vi "2022_version.vi"() -> ()   [LabVIEW 2022 SP3]
panel:
  out "output cluster":cluster{"current speed":dbl, "command":string}
  in  "input":cluster{"current speed":dbl, "command":string}
  out "test pic":picture
  in  "image_path":path
  out "return value":string
  in  "module path":path
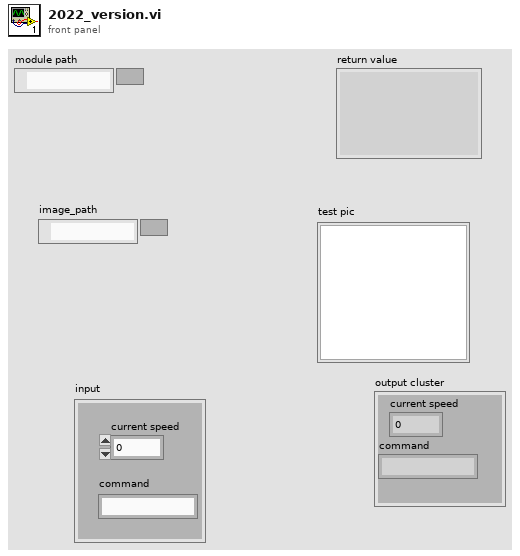
[diagram p1: front panel]
types:
  T1 = typedef "imagedata.ctl" = cluster{"image type":i32, "image depth":i32, "image":u8[], "mask":u8[], "colors":u32[], "Rectangle":cluster{"left":i16, "top":i16, "right":i16, "bottom":i16}}
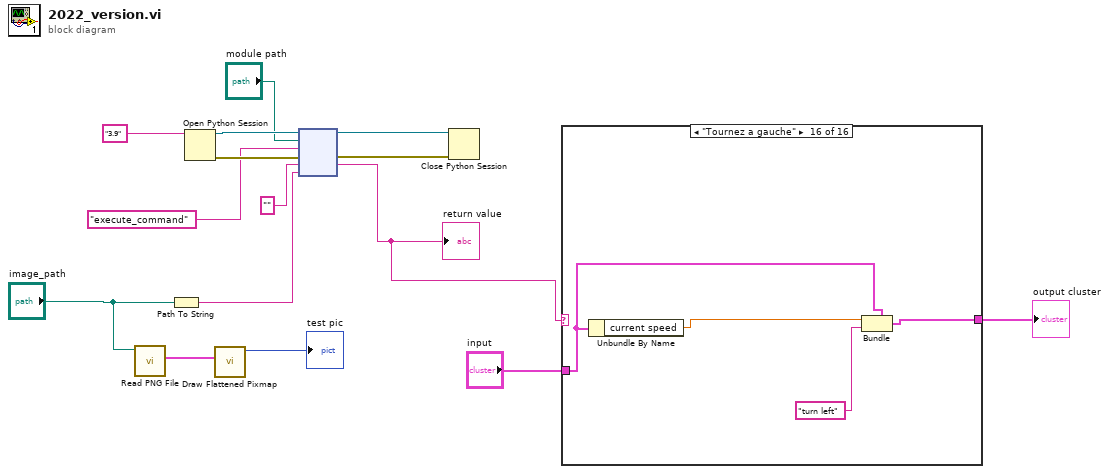
[diagram p0: block diagram]
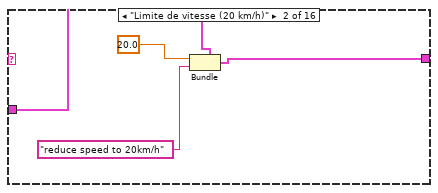
[diagram p3: hidden frame]
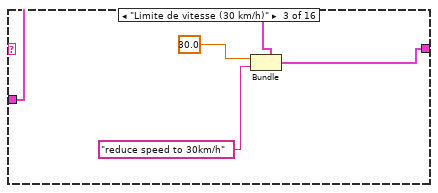
[diagram p4: hidden frame]
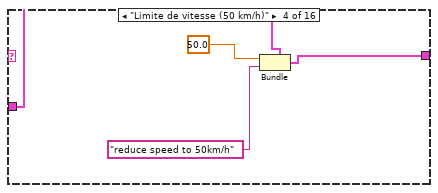
[diagram p5: hidden frame]
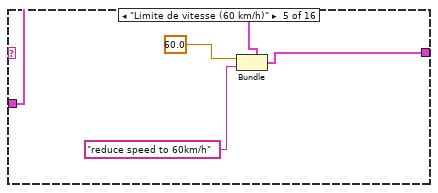
[diagram p6: hidden frame]
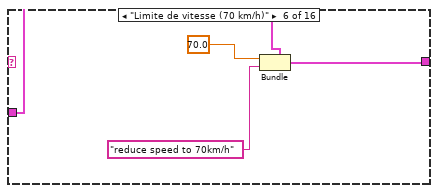
[diagram p7: hidden frame]
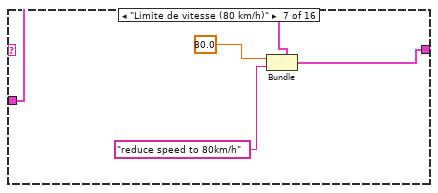
[diagram p8: hidden frame]
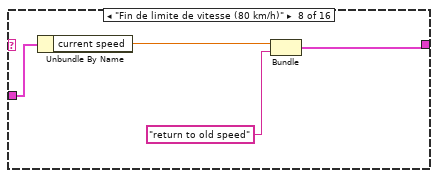
[diagram p9: hidden frame]
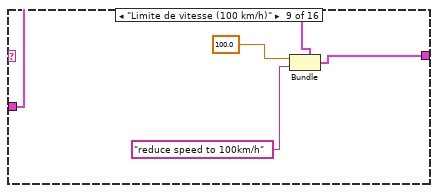
[diagram p10: hidden frame]
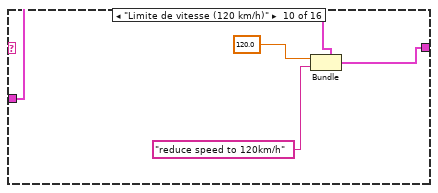
[diagram p11: hidden frame]
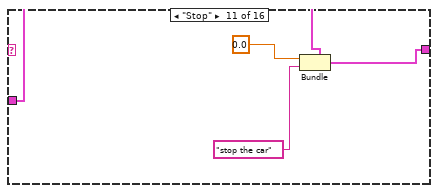
[diagram p12: hidden frame]
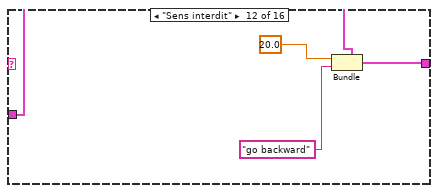
[diagram p13: hidden frame]
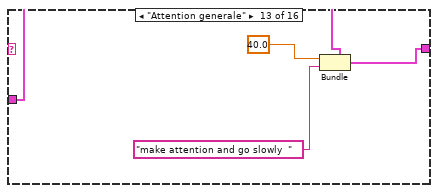
[diagram p14: hidden frame]
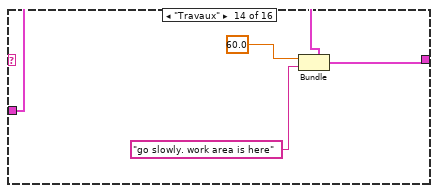
[diagram p15: hidden frame]
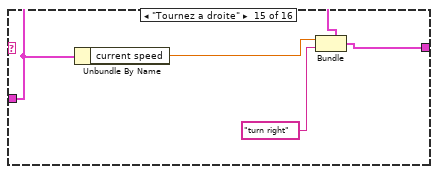
[diagram p16: hidden frame]
diagram:
  n1 = call <vilib>:"Read PNG File.vi"("path to PNG file"="image_path") -> ("image data"=w5:T1)  [unwired: 8 in, 2 out]
  n2 = Path To String(path="image_path") -> (string=w7:string)
  n3 = Open Python Session(python version="3.9" ("Python version")) -> (session out=w15:refnum<k35>, error out=w13:errorcluster)  [unwired: 2 in]
  n4 = call <vilib>:"Draw Flattened Pixmap.vi"("image data"=w5) -> ("new picture"=→"test pic":picture)  [unwired: 8 in]
  n5 = node(w15, "module path", "execute_command" ("function name"), w13, "", w7) -> (w14:refnum<k35>, w12:errorcluster, w3:string)  [unwired: 1 in, 2 out]
  "return value" <- w3
  n6 = Close Python Session(session in=w14, error in=w12) -> ()  [unwired: 1 out]
  n7 = case shown="\"Tournez a gauche\"" w3 {
    tunnel: "input" -> [w16 w20 w22 w26 w30 w34 w38 w43 w46 w49 w54 w58 w62 w66 w70 w74]
    tunnel: [w16 w17 w21 w25 w29 w33 w37 w41 w45 w50 w53 w57 w61 w65 w71 w75] -> w1
    frame "False", Default {
    }
    frame "Limite de vitesse (20 km/h)" {
      n8 = Bundle(cluster=w20, "current speed"=20.0, "command"="reduce speed to 20km/h") -> (w17:cluster{"current speed":dbl, "command":string})
    }
    frame "Limite de vitesse (30 km/h)" {
      n9 = Bundle(cluster=w22, "current speed"=30.0, "command"="reduce speed to 30km/h") -> (w21:cluster{"current speed":dbl, "command":string})
    }
    frame "Limite de vitesse (50 km/h)" {
      n10 = Bundle(cluster=w26, "current speed"=50.0, "command"="reduce speed to 50km/h") -> (w25:cluster{"current speed":dbl, "command":string})
    }
    frame "Limite de vitesse (60 km/h)" {
      n11 = Bundle(cluster=w30, "current speed"=60.0, "command"="reduce speed to 60km/h") -> (w29:cluster{"current speed":dbl, "command":string})
    }
    frame "Limite de vitesse (70 km/h)" {
      n12 = Bundle(cluster=w34, "current speed"=70.0, "command"="reduce speed to 70km/h") -> (w33:cluster{"current speed":dbl, "command":string})
    }
    frame "Limite de vitesse (80 km/h)" {
      n13 = Bundle(cluster=w38, "current speed"=80.0, "command"="reduce speed to 80km/h") -> (w37:cluster{"current speed":dbl, "command":string})
    }
    frame "Fin de limite de vitesse (80 km/h)" {
      n14 = Unbundle By Name(w43) -> ("current speed"=w42:dbl)
      n15 = Bundle("current speed"=w42, "command"="return to old speed") -> (w41:cluster{"current speed":dbl, "command":string})  [unwired: 1 in]
    }
    frame "Limite de vitesse (100 km/h)" {
      n16 = Bundle(cluster=w46, "current speed"=100.0, "command"="reduce speed to 100km/h") -> (w45:cluster{"current speed":dbl, "command":string})
    }
    frame "Limite de vitesse (120 km/h)" {
      n17 = Bundle(cluster=w49, "current speed"=120.0, "command"="reduce speed to 120km/h") -> (w50:cluster{"current speed":dbl, "command":string})
    }
    frame "Stop" {
      n18 = Bundle(cluster=w54, "current speed"=0.0, "command"="stop the car") -> (w53:cluster{"current speed":dbl, "command":string})
    }
    frame "Sens interdit" {
      n19 = Bundle(cluster=w58, "current speed"=20.0, "command"="go backward") -> (w57:cluster{"current speed":dbl, "command":string})
    }
    frame "Attention generale" {
      n20 = Bundle(cluster=w62, "current speed"=40.0, "command"="make attention and go slowly  ") -> (w61:cluster{"current speed":dbl, "command":string})
    }
    frame "Travaux" {
      n21 = Bundle(cluster=w66, "current speed"=60.0, "command"="go slowly. work area is here") -> (w65:cluster{"current speed":dbl, "command":string})
    }
    frame "Tournez a droite" {
      n22 = Unbundle By Name(w70) -> ("current speed"=w69:dbl)
      n23 = Bundle(cluster=w70, "current speed"=w69, "command"="turn right") -> (w71:cluster{"current speed":dbl, "command":string})
    }
    frame "Tournez a gauche" {
      n24 = Unbundle By Name(w74) -> ("current speed"=w73:dbl)
      n25 = Bundle(cluster=w74, "current speed"=w73, "command"="turn left") -> (w75:cluster{"current speed":dbl, "command":string})
    }
  }
  "output cluster" <- w1
